vi "GetEnvironmentalInfo.vi"() -> (0 "Environmental Info":T1)   [LabVIEW 2015]
uses:
  TCSLINK_global.vi
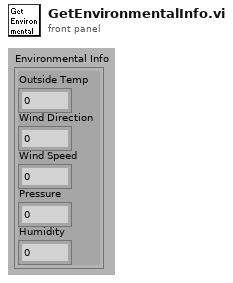
[diagram p1: front panel]
types:
  T1 = cluster{"Outside Temp":dbl, "Wind Direction":dbl, "Wind Speed":dbl, "Pressure":dbl, "Humidity":dbl}
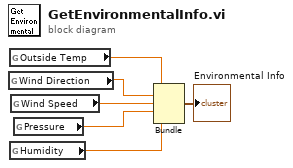
[diagram p0: block diagram]
diagram:
  n1 = global read "TCSLINK_global.vi" "Wind Direction"() -> (w4:dbl)
  n2 = global read "TCSLINK_global.vi" "Outside Temp"() -> (w5:dbl)
  n3 = global read "TCSLINK_global.vi" "Humidity"() -> (w2:dbl)
  n4 = global read "TCSLINK_global.vi" "Wind Speed"() -> (w6:dbl)
  n5 = global read "TCSLINK_global.vi" "Pressure"() -> (w3:dbl)
  n6 = Bundle("Outside Temp"=w5, "Wind Direction"=w4, "Wind Speed"=w6, "Pressure"=w3, "Humidity"=w2) -> (→"Environmental Info":T1)  [unwired: 1 in]
